vi "Open gRPC Server-Client [2] - Code Generator.vi"   [LabVIEW 2024]
panel:
  # "Open gRPC Server-Client[2] - Code Generator..."
types:
  T1 = enum32{"Invalid", "Standard", "Closed", "Hidden", "Minimized", "Maximized"}
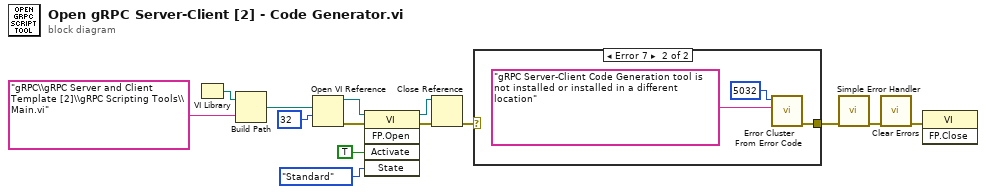
[diagram p0: block diagram]
diagram:
  n1 = VI Library() -> (path=w14:path)
  n2 = Build Path(base path=w14, name or relative path="gRPC\\gRPC Server and Client Template [2]\\gRPC Scripting Tools\\Main.vi") -> (appended path=w5:path)
  n3 = Open VI Reference(vi path=w5, options=32) -> (vi reference=w11:refnum<vi>, error out=w10:errorcluster)  [unwired: 4 in]
  n4 = invoke class="VI" method="FP.Open"(reference=w11, error in=w10, "Activate"=TRUE ("Activate?"), "State"=T1."Standard") -> (reference out=w6:refnum<vi>, error out=w7:errorcluster)  [unwired: 1 in, 3 out]
  n5 = Close Reference(reference=w6, error in (no error)=w7) -> (error out=w4:errorcluster)
  n6 = case shown="Error 7" w4 {
    selector: w4 -> [w15 _]
    tunnel: [w15 w16] -> w3
    frame #0 {
    }
    frame #1 {
      n7 = call <vilib>:"Error Cluster From Error Code.vi"("error message (\"\")"="gRPC Server-Client Code Generation tool is not installed or installed in a different location" ("error message (\"\")"), "error code (0)"=5032) -> ("error out"=w16:errorcluster)  [unwired: 7 in]
    }
  }
  n8 = call <vilib>:"Simple Error Handler.vi"("error in (no error)"=w3) -> ("error out"=w2:errorcluster)  [unwired: 4 in, 4 out]
  n9 = call <vilib>:"Clear Errors.vi"("error in (no error)"=w2) -> ("error out"=w1:errorcluster)  [unwired: 5 in, 1 out]
  n10 = invoke class="VI" method="FP.Close"(error in=w1) -> ()  [unwired: 2 in, 3 out]
